vi "DataArrangement(ID).vi"(8 "error in (no error)":errorcluster, 9 "y":i32, 10 "ID":i32[](array[numeric]), 11 "InputData":dbl[](array[numeric])) -> (0 "error out":errorcluster, 3 "OutputData":dbl[](array[numeric]))   [LabVIEW 2019, in "Zen Analytics.lvlib" / "Zen Analytics.lvclass"]
uses:
  Zen Analytics.lvclass
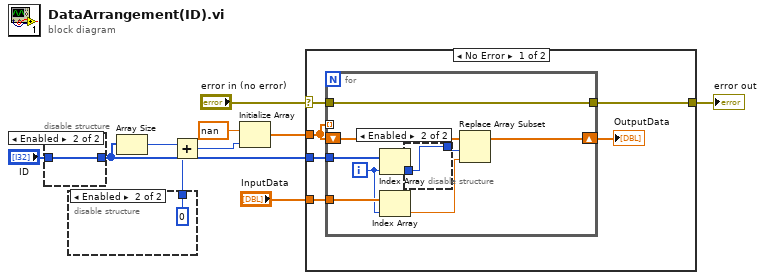
[diagram p0: block diagram]
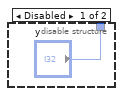
[diagram p2: hidden frame]
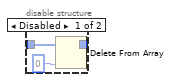
[diagram p3: hidden frame]
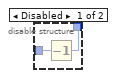
[diagram p4: hidden frame]
diagram:
  n1 = disable-structure shown="Enabled" {
    disable-tunnel: "ID" -> [w13 w14]
    disable-tunnel: [w11 w14] -> w4
    frame Disabled {
      n2 = Delete From Array(array=w13, index=0) -> (array with subset deleted=w11:i32[])  [unwired: 1 in, 1 out]
    }
    frame Enabled {
    }
  }
  n3 = disable-structure shown="Enabled" {
    disable-tunnel: ["y" 0 ("y")] -> w1
    frame Disabled {
    }
    frame Enabled {
    }
  }
  n4 = Array Size(array=w4) -> (size(s)=w3:i32)
  n5 = Add(x=w3, y=w1) -> (x+y=w2:i32)
  n6 = Initialize Array(nan ("element"), w2) -> (w7:dbl[])
  n7 = case shown="No Error" "error in (no error)" {
    selector: "error in (no error)" -> [w20 w35]
    tunnel: [w21 w35] -> w9
    tunnel: w7 -> [w17 _]
    tunnel: "InputData" -> [w19 _]
    tunnel: w4 -> [w18 _]
    frame No Error {
      n8 = for {
        tunnel: w19 -> [w28]
        tunnel: w18 -> [w24]
        shift-right: [w30] -> w22
        shift-left: w17 -> [w31]
        tunnel: [w29] -> w21
        tunnel: w20 -> [w29]
        tunnel: w17 -> [_] mode=indexing
        i -> [w25]
        n9 = Index Array(array=w24, index=w25) -> (element=w23:i32)
        n10 = Index Array(array=w28, index=w25) -> (element=w26:dbl)
        n11 = disable-structure shown="Enabled" {
          disable-tunnel: [w33 w34] -> w27
          disable-tunnel: w23 -> [w32 w34]
          frame Disabled {
            n12 = Decrement(x=w32) -> (x-1=w33:i32)
          }
          frame Enabled {
          }
        }
        n13 = Replace Array Subset "Replace Array Subset"(array=w31, new element=w26, index=w27) -> (w30:dbl[])
      }
      "OutputData" <- w22
    }
    frame Error {
    }
  }
  "error out" <- w9
